vi "TSCAN_DBCTree.vi"(9 "子节点":string[][](array[string]), 10 "父节点":string[](array[string]), 11 "控件":refnum<vi>) -> ()   [LabVIEW 2019]
panel:
  out "活动项:标识符":string
  in  "树形控件":string(tree)
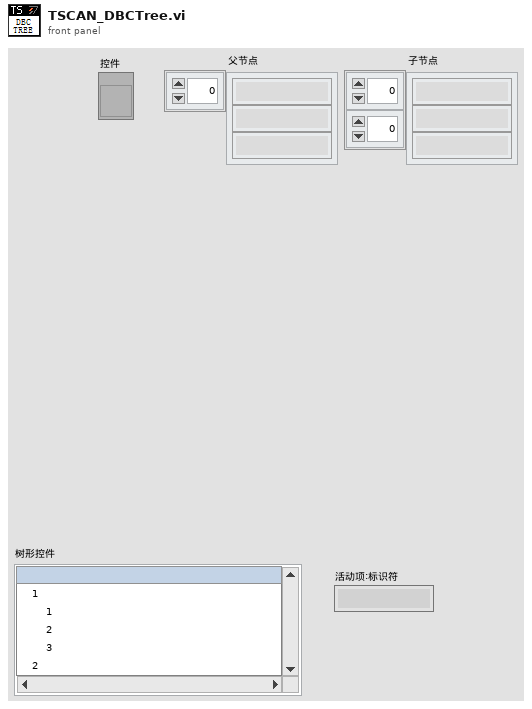
[diagram p1: front panel]
types:
  T1 = typedef "LVPoint32TypeDef.ctl" = cluster{"Horizontal":i32, "Vertical":i32}
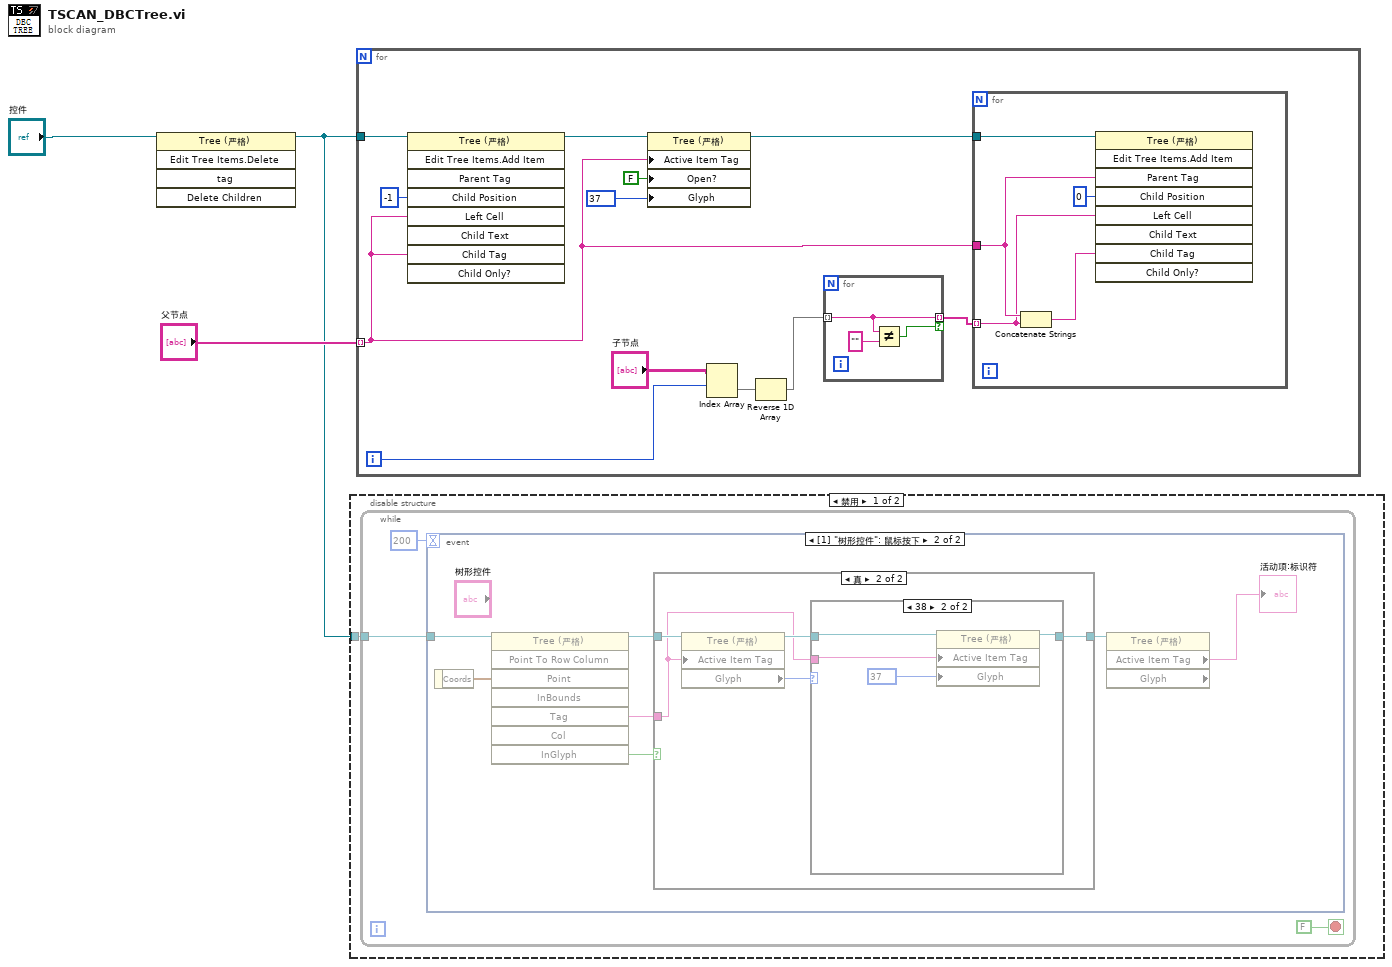
[diagram p0: block diagram]
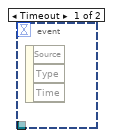
[diagram p2: hidden frame]
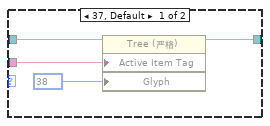
[diagram p4: hidden frame]
diagram:
  n1 = invoke class="Tree (严格)" method="Edit Tree Items.Delete"(reference="控件") -> (reference out=w2:refnum<vi>)  [unwired: 4 in, 4 out]
  n2 = disable-structure shown="禁用" {
    disable-tunnel: w2 -> [w4 _]
    frame Disabled {
      n3 = while {
        tunnel: w4 -> [w5]
        stop <- FALSE stop-if-true
        n4 = event shown="[1] \"树形控件\": 鼠标按下" {
          selector: _ -> [_ _]
          dyn-events: _ -> [_ _]
          timeout: 200 -> [_ _]
          tunnel: w5 -> [_ w13]
          event Timeout {
            n5 = event-data() -> ()  [unwired: 1 in, 3 out]
          }
          event "树形控件": Mouse Down {
            n6 = event-data() -> ("Coords"=w14:T1)  [unwired: 1 in]
            n7 = invoke class="Tree (严格)" method="Point To Row Column"(reference=w13, "Point"=w14) -> (reference out=w10:refnum<vi>, "Tag"=w11:string, "InGlyph"=w12:bool)  [unwired: 6 in, 5 out]
            n8 = case shown="真" w12 {
              tunnel: w11 -> [_ w17]
              tunnel: w10 -> [w15 w20]
              tunnel: [w15 w16] -> w9
              frame False {
              }
              frame True {
                n9 = property class="Tree (严格)"(reference=w20, "Active Item Tag"=w17) -> (reference out=w18:refnum<vi>, "Glyph"=w19:i32)  [unwired: 1 in, 1 out]
                n10 = case shown="38" w19 {
                  tunnel: w18 -> [w23 w27]
                  tunnel: w17 -> [w22 w26]
                  tunnel: [w21 w25] -> w16
                  frame 37, Default {
                    n11 = property class="Tree (严格)"(reference=w23, "Active Item Tag"=w22, "Glyph"=38) -> (reference out=w21:refnum<vi>)  [unwired: 1 in, 1 out]
                  }
                  frame 38 {
                    n12 = property class="Tree (严格)"(reference=w27, "Active Item Tag"=w26, "Glyph"=37) -> (reference out=w25:refnum<vi>)  [unwired: 1 in, 1 out]
                  }
                }
              }
            }
            n13 = property class="Tree (严格)" props=["Active Item Tag", "Glyph"](reference=w9) -> ("Active Item Tag"=→"活动项:标识符":string)  [unwired: 1 in, 3 out]
          }
        }
      }
    }
    frame Enabled {
    }
  }
  n14 = for {
    tunnel: "父节点" -> [w34] mode=indexing
    tunnel: w2 -> [w40]
    i -> [w32]
    n15 = invoke class="Tree (严格)" method="Edit Tree Items.Add Item"(reference=w40, "Child Position"=-1 ("子项位置"), "Left Cell"=w34, "Child Tag"=w34) -> (reference out=w39:refnum<vi>)  [unwired: 5 in, 8 out]
    n16 = property class="Tree (严格)"(reference=w39, "Active Item Tag"=w34, "Open?"=FALSE ("活动项:打开？"), "Glyph"=37) -> (reference out=w36:refnum<vi>)  [unwired: 1 in, 1 out]
    n17 = Index Array(array="子节点", index (row)=w32) -> (element=w31:string[])  [unwired: 1 in]
    n18 = Reverse 1D Array(array=w31) -> (reversed array=w30:string[])
    n19 = for {
      tunnel: w30 -> [w43] mode=indexing
      tunnel: [w43] -> w29 mode=indexing if=w41
      n20 = Not Equal?(x=w43, y="") -> (x != y?=w41:bool)
    }
    n21 = for {
      tunnel: w36 -> [w48]
      tunnel: w29 -> [w44] mode=indexing
      tunnel: w34 -> [w46]
      n22 = Concatenate Strings(w46, w44) -> (w45:string)
      n23 = invoke class="Tree (严格)" method="Edit Tree Items.Add Item"(reference=w48, "Parent Tag"=w46, "Child Position"=0 ("子项位置"), "Left Cell"=w44, "Child Tag"=w45) -> ()  [unwired: 4 in, 9 out]
    }
  }
